vi "Add Extensions to Web Service.vi"(8 "error in (no error)":errorcluster, 11 "Project":path=path "P:/alsmith/Sales/users/ACS/LabVIEW Continuous Integration/Core/LabVIEW CI Service/LabVIEW CI Service.lvproj") -> (0 "error out":errorcluster)   [LabVIEW 2014]
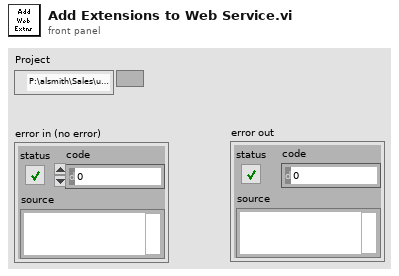
[diagram p1: front panel]
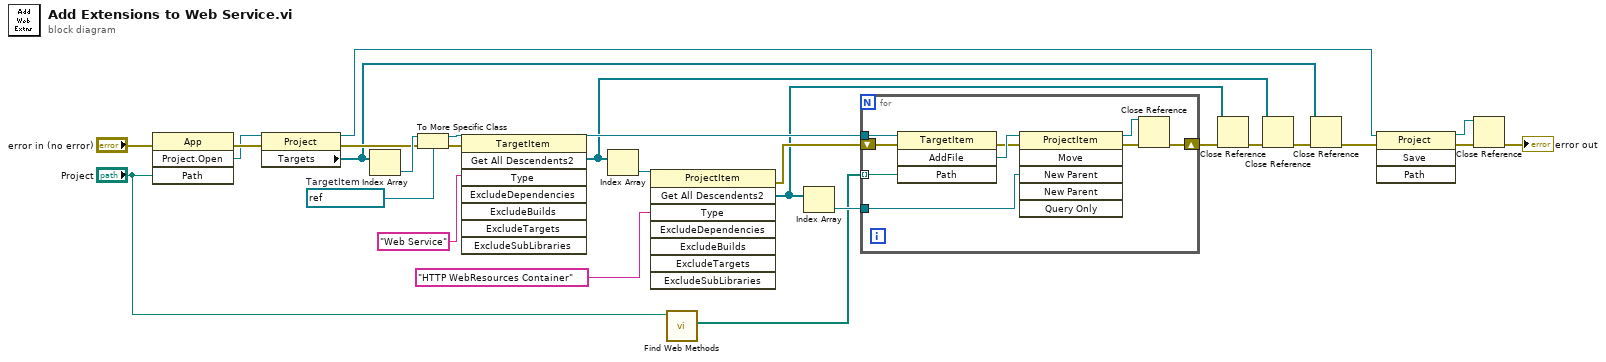
[diagram p0: block diagram]
diagram:
  w27 = refnum<vi> refnum  # TargetItem
  n1 = invoke class="App" method="Project.Open"(error in="error in (no error)", "Path"="Project") -> (error out=w25:errorcluster, "Project:Open"=w21:refnum<vi>)  [unwired: 2 in, 2 out]
  n2 = property class="Project"(reference=w21, error in=w25) -> (reference out=w18:refnum<vi>, error out=w24:errorcluster, "Targets"=w6:refnum<vi>[])
  n3 = Index Array(array=w6) -> (element=w26:refnum<vi>)  [unwired: 1 in]
  n4 = To More Specific Class(target class=w27, reference=w26, error in=w24) -> (specific class reference=w20:refnum<vi>, error out=w23:errorcluster)
  n5 = invoke class="TargetItem" method="Get All Descendents2"(reference=w20, error in=w23, "Type"="Web Service") -> (reference out=w15:refnum<vi>, "Get All Descendents2"=w7:refnum<vi>[])  [unwired: 5 in, 6 out]
  n6 = Index Array(array=w7) -> (element=w17:refnum<vi>)  [unwired: 1 in]
  n7 = invoke class="ProjectItem" method="Get All Descendents2"(reference=w17, "Type"="HTTP WebResources Container" ("Type String")) -> (error out=w14:errorcluster, "Get All Descendents2"=w8:refnum<vi>[])  [unwired: 6 in, 6 out]
  n8 = call "Find Web Methods.vi"("Project"="Project") -> ("Web Methods"=w4:path[])  [unwired: 10 in]
  n9 = Index Array(array=w8) -> (element=w13:refnum<vi>)  [unwired: 1 in]
  n10 = for {
    tunnel: w15 -> [w36]
    tunnel: w13 -> [w32]
    shift-right: [w31] -> w10
    shift-left: w14 -> [w35]
    tunnel: w4 -> [w28] mode=indexing
    n11 = invoke class="TargetItem" method="AddFile"(reference=w36, error in=w35, "Path"=w28) -> (error out=w29:errorcluster, "AddFile"=w33:refnum<vi>)  [unwired: 1 in, 2 out]
    n12 = invoke class="ProjectItem" method="Move"(reference=w33, error in=w29, "New Parent"=w32) -> (reference out=w30:refnum<vi>, error out=w34:errorcluster)  [unwired: 3 in, 4 out]
    n13 = Close Reference(reference=w30, error in (no error)=w34) -> (error out=w31:errorcluster)
  }
  n14 = Close Reference(reference=w8, error in (no error)=w10) -> (error out=w9:errorcluster)
  n15 = Close Reference(reference=w7, error in (no error)=w9) -> (error out=w3:errorcluster)
  n16 = Close Reference(reference=w6, error in (no error)=w3) -> (error out=w2:errorcluster)
  n17 = invoke class="Project" method="Save"(reference=w18, error in=w2) -> (reference out=w11:refnum<vi>, error out=w16:errorcluster)  [unwired: 2 in, 2 out]
  n18 = Close Reference(reference=w11, error in (no error)=w16) -> (error out=→"error out":errorcluster)
